vi "Goal_set.vi"(8 "error in (no error)":errorcluster, 10 "Goal":cluster{"X":dbl, "Y":dbl}) -> (0 "error out":errorcluster)   [LabVIEW 2009, in "NetworkVarTarget.lvlib"]
uses:
  NetworkVarTarget.lvlib
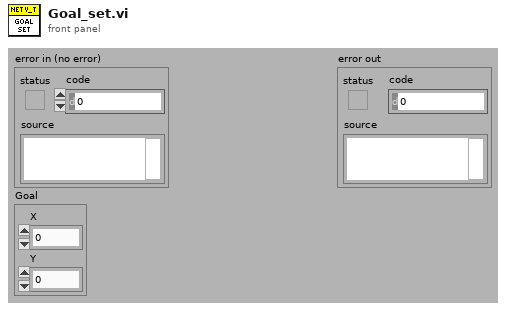
[diagram p1: front panel]
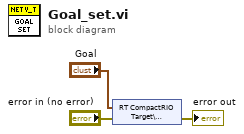
[diagram p0: block diagram]
diagram:
  n1 = shared-variable "RT CompactRIO Target\\NetworkVar.lvlib\\Goal"("Goal", error in="error in (no error)") -> (error out=→"error out":errorcluster)
